vi "User Selected Temperature.vi"(7 "User Selected Temperature":T1, 8 "Error In":errorcluster, 9 "GEA Inputs":T2 {"Destination" format="%.0x"; "Source" format="%.0x"}, 10 "Standalone?":bool, 11 "GEA2 Reference In":refnum<k24>) -> (0 "Error Out":errorcluster, 3 "GEA2 Reference Out":refnum<k24>)   [LabVIEW 2016, in "Centauro.lvlib"]
uses:
  Projects/Centauro.lvlib
  Q:/Common/DLLs/GEA3/GeaCommunication.dll
  Common/DLLs/GEA3/GeaCommunication.dll
  Common/LabVIEW GEA2 Toolkit/LabVIEW_GEA2_Toolkit.lvlibp/type defs/Source_Destination.ctl
  type defs/User Selected Temperature.ctl
  Common/LabVIEW GEA2 Toolkit/LabVIEW_GEA2_Toolkit.lvlibp/type defs/ERD Write Data In.ctl
  Common/LabVIEW GEA2 Toolkit/LabVIEW_GEA2_Toolkit.lvlibp/type defs/Data Type.ctl
  Common/LabVIEW GEA2 Toolkit/LabVIEW_GEA2_Toolkit.lvlibp
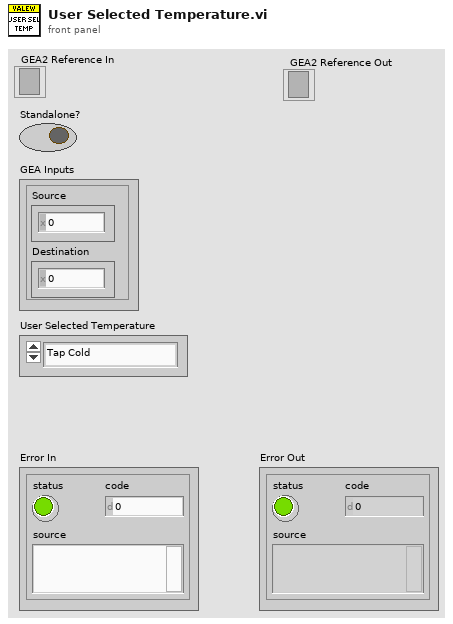
[diagram p1: front panel]
types:
  T1 = typedef "Centauro.lvlib/User Selected Temperature.ctl" = enum16{"Tap Cold", "Cold", "Cool", "Colors", "Warm", "Hot"}
  T2 = typedef "LabVIEW_GEA2_Toolkit.lvlibp/Source_Destination.ctl" = cluster{"Source":u8, "Destination":u8}
  T3 = typedef "LabVIEW_GEA2_Toolkit.lvlibp/ERD Write Data In.ctl" = cluster{"ERD Number":u16, "Data Type":T4, "Data":string}
  T4 = typedef "LabVIEW_GEA2_Toolkit.lvlibp/Data Type.ctl" = enum16{"string", "boolean", "uint8_t", "uint16_t", "uint32_t", "uint64_t", "int8_t", "int16_t", "int32_t", "int64_t"}
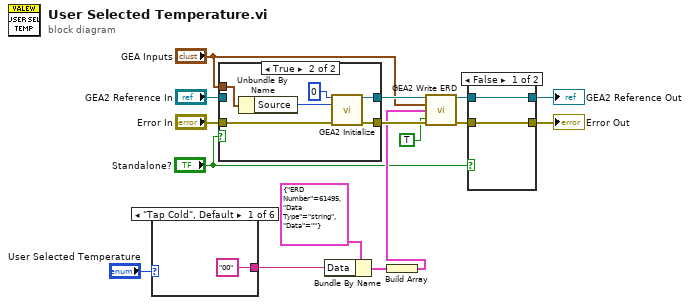
[diagram p0: block diagram]
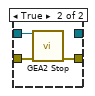
[diagram p2: hidden frame]
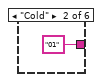
[diagram p4: hidden frame]
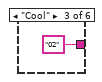
[diagram p5: hidden frame]
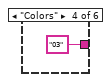
[diagram p6: hidden frame]
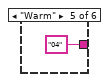
[diagram p7: hidden frame]
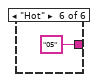
[diagram p8: hidden frame]
diagram:
  n1 = case shown="\"Tap Cold\", Default" "User Selected Temperature" {
    tunnel: ["00" "01" "02" "03" "04" "05"] -> w6
    frame "Tap Cold", Default {
    }
    frame "Cold" {
    }
    frame "Cool" {
    }
    frame "Colors" {
    }
    frame "Warm" {
    }
    frame "Hot" {
    }
  }
  n2 = case shown="True" "Standalone?" {
    tunnel: "Error In" -> [w23 w30]
    tunnel: [w23 w29] -> w16
    tunnel: "GEA2 Reference In" -> [w24 _]
    tunnel: [w24 w28] -> w11
    tunnel: "GEA Inputs" -> [_ w26]
    frame False {
    }
    frame True {
      n3 = Unbundle By Name(w26) -> ("Source"=w27:u8)
      n4 = call "GEA2 Initialize.vi"("Board Index"=0, "Source Address"=w27, "error in"=w30) -> ("GEA2 Reference Out"=w28:refnum<k24>, "error out"=w29:errorcluster)  [unwired: 10 in, 1 out]
    }
  }
  n5 = Bundle By Name(cluster=T3 {"ERD Number"=61495, "Data Type"=enum."string", "Data"=""} ("ERD Write Data In"), "Data"=w6) -> (w8:T3)
  n6 = Build Array(w8) -> (w7:T3[])
  n7 = call "GEA2 Write ERD.vi"("GEA2 Reference In"=w11, "GEA Inputs"="GEA Inputs", "Write ERD List"=w7, "Error In"=w16, "Verify ERD Response?"=TRUE) -> ("GEA2 Reference Out"=w2:refnum<k24>, "Error Out"=w1:errorcluster)  [unwired: 8 in, 1 out]
  n8 = case shown="False" "Standalone?" {
    tunnel: w1 -> [w31 w35]
    tunnel: [w31 w34] -> w14
    tunnel: w2 -> [w32 w33]
    tunnel: [w32 _] -> w12
    frame False {
    }
    frame True {
      n9 = call "GEA2 Stop.vi"("GEA2 Reference In"=w33, "Error In"=w35) -> ("Error Out"=w34:errorcluster)  [unwired: 13 in]
    }
  }
  "Error Out" <- w14
  "GEA2 Reference Out" <- w12
